vi "Write packed data to DRAM.vi"(2 "Write DRAM enable?":bool) -> (7 "Write DRAM done?":bool)   [LabVIEW 2015]
uses:
  <vilib>/Platform/TimedLoop/XDataNode/wakeup.ctl
  <vilib>/Platform/TimedLoop/XDataNode/XDNodeRunTimeDep.lvlib
  <vilib>/Platform/TimedLoop/XDataNode/nitl_modes.ctl
  <vilib>/Platform/TimedLoop/XDataNode/timing_clust.ctl
  <vilib>/Platform/TimedLoop/XDataNode/XDataNode.xnode
  <vilib>/rvi/DataTransferAndStorage/Container/XNode/niFpgaContainer.xnode
  <vilib>/rvi/interface/RandomDataEmulation/nirviRandomDataFpgaReadWriteTemplate.vi
  <vilib>/rvi/Memory/Memory_Emulation/niFpgaMemoryFastEmulationDramWriteAndRequestData.vi
  <vilib>/rvi/Memory/Memory_Emulation/niFpgaMemoryEmulationDramWriteAndRequestData.vi
  <vilib>/rvi/Memory/Memory_Emulation/niFpgaMemoryEmulationDramRetrieveData.vi
panel:
  out "unpacked data readed":i32
  out "Read DRAM address":u32
  out "Write DRAM address":u32
  in  "Total elements to write":i32
  out "read DRAM done?":bool
  in  "Total packed data to write?":u32
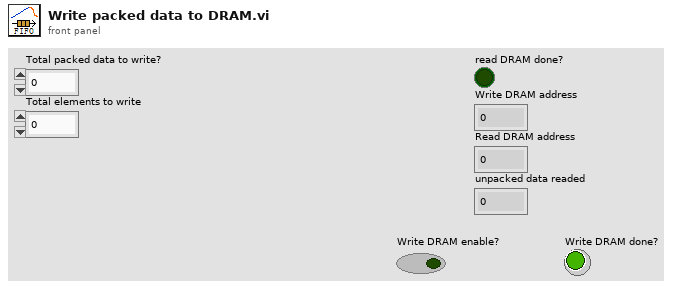
[diagram p1: front panel]
types:
  T1 = enum16{"Wait on Trigger", "Write DRAM", "Read DRAM"}
  T2 = typedef "XDNodeRunTimeDep.lvlib/timing_clust.ctl" = cluster{"Expected End [f-1]":u64, "Actual End [f-1]":u64, "Finished Late? [f-1]":bool, "Expected End [i-1]":u64, "Actual End [i-1]":u64, "Finished Late? [i-1]":bool, "Expected Start [i]":u64, "Actual Start [i]":u64, "Expected Start [f]":u64, "Actual Start [f]":u64, "Source Name":string, "Structure Name":string, "Period":i64, "Deadline":i64, "Offset":i64, "Start":i64, "Priority":i32, "Timeout":i32, "Mode":T3, "Wakeup Reason":T4, "Error":errorcluster, "Source Type":string, "Secondary Source Type":string, "Global End Time":u64, "Global Start Time":u64, "Frame Duration":u64, "Iteration Duration":u64, "Assigned CPU":i32, "I/O Scan Engine Mode":u32}
  T3 = typedef "XDNodeRunTimeDep.lvlib/nitl_modes.ctl" = enum32{"No Change", "Process missed periods, maintain original phase", "Discard missed periods, maintain original phase", "Process missed periods, ignore original phase", "Discard missed periods, ignore original phase"}
  T4 = typedef "XDNodeRunTimeDep.lvlib/wakeup.ctl" = enum32{"Normal", "Aborted", "Asynchronous wakeup", "Timing source error", "Timed loop error", "Timeout"}
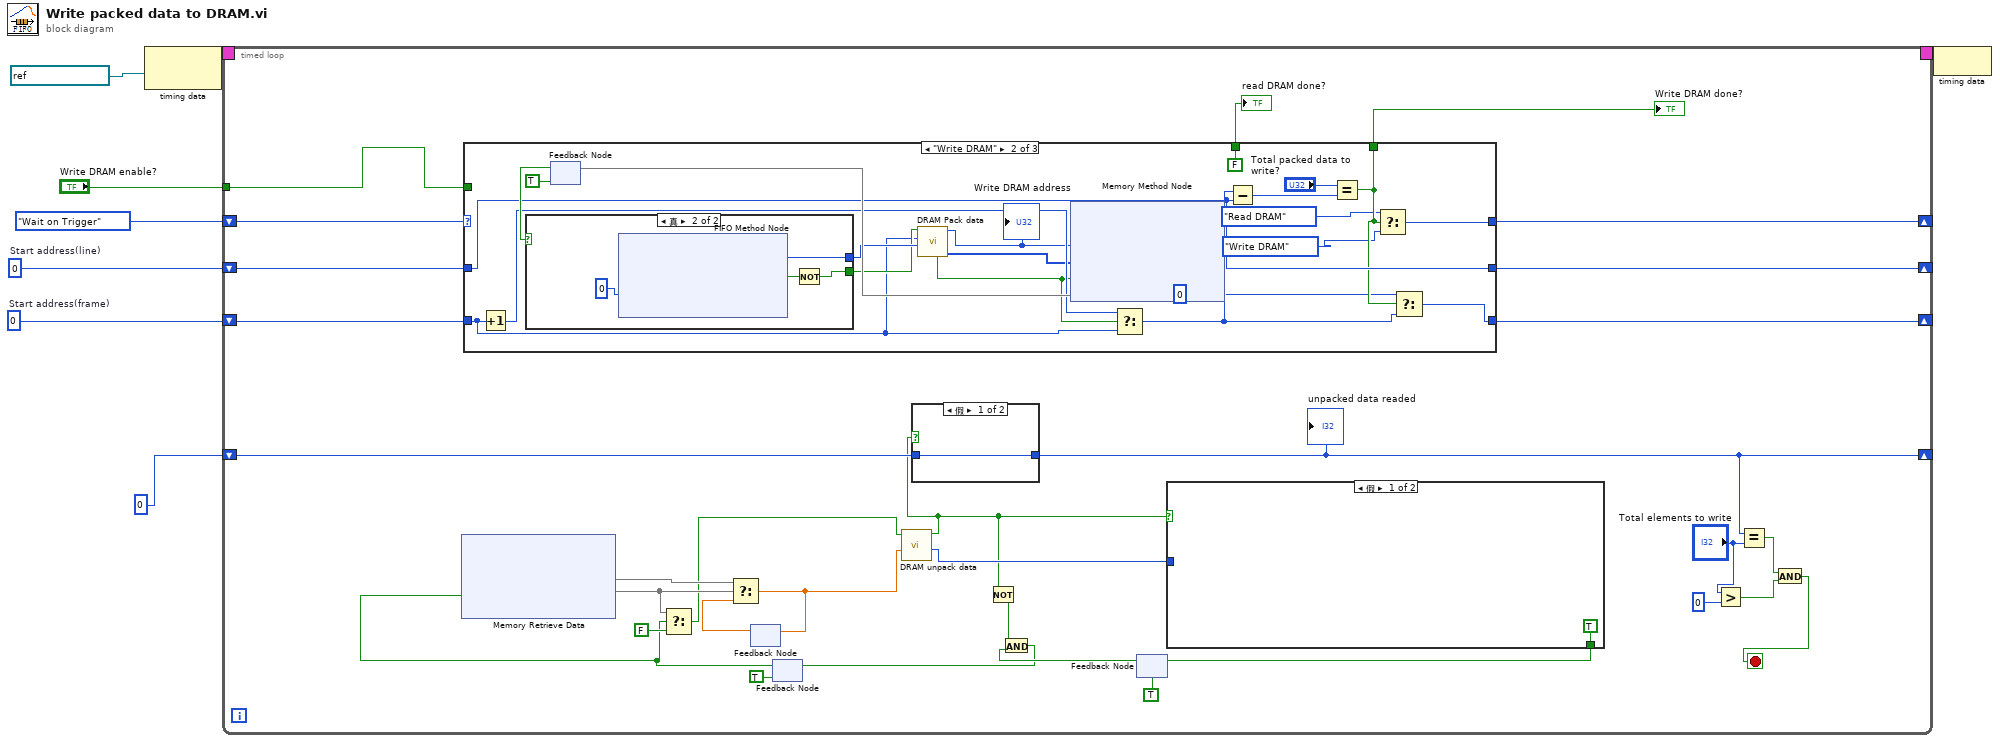
[diagram p0: block diagram]
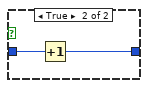
[diagram p2: hidden frame]
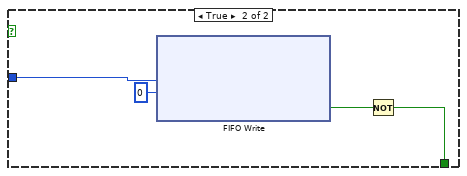
[diagram p3: hidden frame]
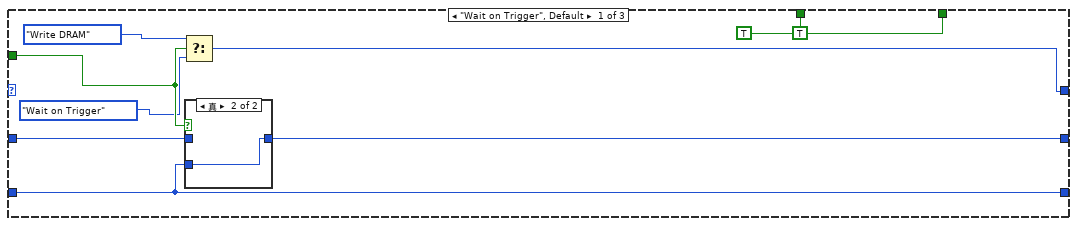
[diagram p4: hidden frame]
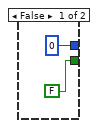
[diagram p6: hidden frame]
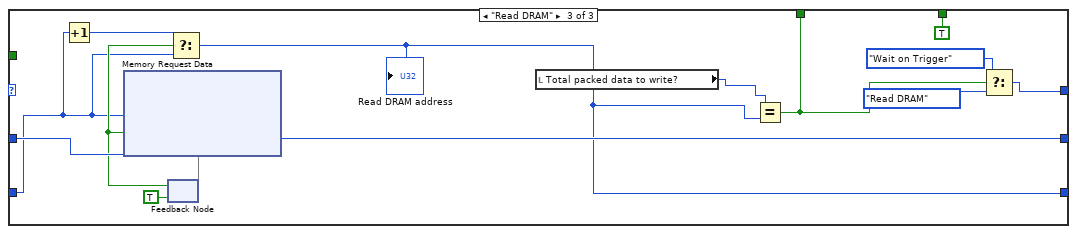
[diagram p7: hidden frame]
diagram:
  w5 = u32 0  # Start address(line)
  w6 = u32 0  # Start address(frame)
  n1 = node-c288(refnum<k21> "DRAM Clock" ("Source Name")) -> (w8:T2)
  n2 = timed-loop {
    timing: w8 -> [_]
    timing-out: [_] -> w7
    shift-right: [w37] -> _
    shift-left: T1."Wait on Trigger" -> [w34]
    shift-right: [w36] -> _
    shift-left: w5 -> [w39]
    shift-right: [w35] -> _
    shift-left: w6 -> [w38]
    tunnel: "Write DRAM enable?" -> [w9]
    shift-right: [w17] -> _
    shift-left: 0 ("Timeout") -> [w19]
    stop <- w11 stop-if-true
    n3 = case shown="\"Write DRAM\"" w34 {
      tunnel: w38 -> [w55 w60 w92]
      tunnel: [w55 w68 w91] -> w35
      tunnel: [w56 w76 w87] -> w37
      tunnel: w39 -> [w54 w74 w97]
      tunnel: [w53 w74 w97] -> w36
      tunnel: [TRUE w71 TRUE] -> w10
      tunnel: w9 -> [w51 _ _]
      tunnel: [TRUE FALSE w86] -> w27
      frame "Wait on Trigger", Default {
        n4 = Select(t=T1."Write DRAM", s=w51, f=T1."Wait on Trigger") -> (s? t:f=w56:T1)
        n5 = case shown="真" w51 {
          tunnel: w55 -> [_ w58]
          tunnel: w54 -> [w57 _]
          tunnel: [w57 w58] -> w53
          frame False {
          }
          frame True {
          }
        }
      }
      frame "Write DRAM" {
        n6 = Increment(x=w60) -> (x+1=w77:u32)
        n7 = feedback #1(TRUE ("Ready for Input")) -> (w78:bool)
        n8 = case shown="真" w78 {
          tunnel: [FALSE w83] -> w62
          tunnel: [u32 0 ("Element") w82] -> w65
          frame False {
          }
          frame True {
            n9 = xnode ("FIFO Method Node")("超时"=0 ("Timeout")) -> ("元素"=w82:u32, "超时？"=w84:bool)  [unwired: 1 in, 1 out]
            n10 = Not(x=w84) -> (.not. x?=w83:bool)
          }
        }
        n11 = call "DRAM Pack data.vi"("Data input"=w65, "Adress input"=w60, "Input valid?"=w62) -> ("Array"=w64:u32[], "Address output"=w63:u32, "output"=w61:bool)  [unwired: 6 in]
        "Write DRAM address" <- w63
        n12 = xnode ("Memory Method Node")("地址"=w63, "数据"=w64, "输入有效"=w61) -> ("输入就绪"=w79)  [unwired: 1 in, 1 out]
        n13 = feedback-in #1(w79) -> ()
        n14 = Select(t=w77, s=w61, f=w60) -> (s? t:f=w70:u32)
        n15 = Subtract(x=w70, y=w74) -> (x-y=w75:u32)
        n16 = Equal?(x="Total packed data to write?", y=w75) -> (x = y?=w71:bool)
        n17 = Select(t=T1."Read DRAM", s=w71, f=T1."Write DRAM") -> (s? t:f=w76:T1)
        n18 = Select(t=u32 0, s=w71, f=w70) -> (s? t:f=w68:u32)
      }
      frame "Read DRAM" {
        n19 = Increment(x=w92) -> (x+1=w93:u32)
        n20 = feedback #2(TRUE ("Ready for Input")) -> (w94:bool)
        n21 = xnode ("Memory Request Data")("地址"=w92, "输入有效"=w94) -> ("输入就绪"=w96)  [unwired: 1 in, 1 out]
        n22 = feedback-in #2(w96) -> ()
        n23 = Select(t=w93, s=w94, f=w92) -> (s? t:f=w91:u32)
        "Read DRAM address" <- w91
        n24 = local read "Total packed data to write?"() -> (w90:u32)
        n25 = Equal?(x=w90, y=w91) -> (x = y?=w86:bool)
        n26 = Select(t=T1."Wait on Trigger", s=w86, f=T1."Read DRAM") -> (s? t:f=w87:T1)
      }
    }
    "Write DRAM done?" <- w10
    "read DRAM done?" <- w27
    n27 = feedback #3() -> (w30:dbl)  [unwired: 1 in]
    n28 = feedback #4(TRUE) -> (w20:bool)
    n29 = xnode ("Memory Retrieve Data")("输出就绪"=w20) -> ("数据"=w31, "输出有效"=w29)  [unwired: 1 in, 1 out]
    n30 = Select(t=w29, s=w20, f=FALSE) -> (s? t:f=w26:bool)
    n31 = Select(t=w31, s=w29, f=w30) -> (s? t:f=w25:dbl)
    n32 = feedback-in #3(w25) -> ()
    n33 = call "DRAM unpack data.vi"("packed data in"=w25, "input valid?"=w26) -> ("unpacked data out"=w24:u32, "output valid?"=w18:bool)  [unwired: 8 in]
    n34 = case shown="假" w18 {
      tunnel: w19 -> [w40 w42]
      tunnel: [w40 w41] -> w17
      frame False {
      }
      frame True {
        n35 = Increment(x=w42) -> (x+1=w41:i32)
      }
    }
    "unpacked data readed" <- w17
    n36 = Not(x=w18) -> (.not. x?=w22:bool)
    n37 = feedback #5(TRUE ("Timed Out?")) -> (w23:bool)
    n38 = And(x=w22, y=w23) -> (x .and. y?=w21:bool)
    n39 = feedback-in #4(w21) -> ()
    n40 = case shown="假" w18 {
      tunnel: [TRUE w45] -> w33
      tunnel: w24 -> [_ w44]
      frame False {
      }
      frame True {
        n41 = xnode ("FIFO Write")("元素"=w44, "超时"=0 ("Timeout")) -> ("超时？"=w47:bool)  [unwired: 1 in, 1 out]
        n42 = Not(x=w47) -> (.not. x?=w45:bool)
      }
    }
    n43 = feedback-in #5(w33) -> ()
    n44 = Greater?(x="Total elements to write", y=0) -> (0:w12:bool)
    n45 = Equal?(x=w17, y="Total elements to write") -> (x = y?=w13:bool)
    n46 = And(x=w13, y=w12) -> (x .and. y?=w11:bool)
  }
  n47 = node-c288(w7) -> ()
